vi "MULTTCP2_Setup.vi"(11 "module name":string) -> (0 "multcmd1":string, 1 "cmdq":string, 2 "async notifier name":string, 3 "block notifier":refnum<notifier>, 4 "async notifier":refnum<notifier>, 5 "blockID":string, 6 "cmd notif":refnum<notifier>)   [LabVIEW 2016]
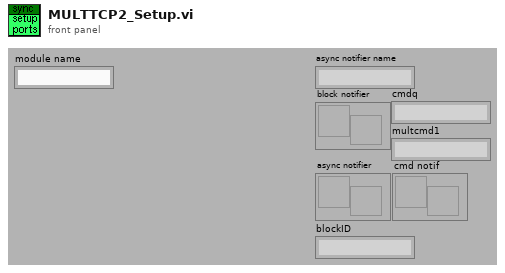
[diagram p1: front panel]
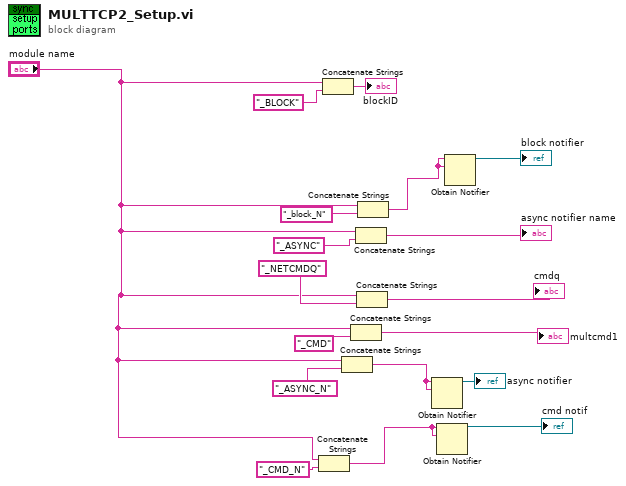
[diagram p0: block diagram]
diagram:
  n1 = Concatenate Strings("module name", "_CMD_N" ("name (unnamed)")) -> (w14:string)
  n2 = Concatenate Strings("module name", "_BLOCK" ("ID")) -> (→"blockID":string)
  n3 = Concatenate Strings("module name", "_ASYNC_N" ("name (unnamed)")) -> (w16:string)
  n4 = Concatenate Strings("module name", "_CMD" ("callerID")) -> (→"multcmd1":string)
  n5 = Concatenate Strings("module name", "_ASYNC" ("callerID")) -> (→"async notifier name":string)
  n6 = Concatenate Strings("module name", "_NETCMDQ" ("messages from socks Q name")) -> (→"cmdq":string)
  n7 = Concatenate Strings("module name", "_block_N" ("name (unnamed)")) -> (w11:string)
  n8 = Obtain Notifier(name (unnamed)=w16, notification data type=w16) -> (notifier out=→"async notifier":refnum<notifier>)  [unwired: 2 in, 2 out]
  n9 = Obtain Notifier(name (unnamed)=w14, notification data type=w14) -> (notifier out=→"cmd notif":refnum<notifier>)  [unwired: 2 in, 2 out]
  n10 = Obtain Notifier(name (unnamed)=w11, notification data type=w11) -> (notifier out=→"block notifier":refnum<notifier>)  [unwired: 2 in, 2 out]
